vi "SBA-5_command case_v2.vi"(6 "Valve control":bool=TRUE, 7 "Case":T1(ring), 8 "error in (no error)":errorcluster, 9 "Val 2":dbl, 10 "Val 1":i32, 11 "VISA resource name":refnum<visa-resource-name>) -> (0 "error out":errorcluster, 1 "bytes out":u32, 2 "StringFromSBA-5":string, 3 "dup VISA resource name":refnum<visa-resource-name>)   [LabVIEW 2016]
uses:
  <vilib>/Instr/_visa.llb/VISA Flush IO Buffer Mask.ctl
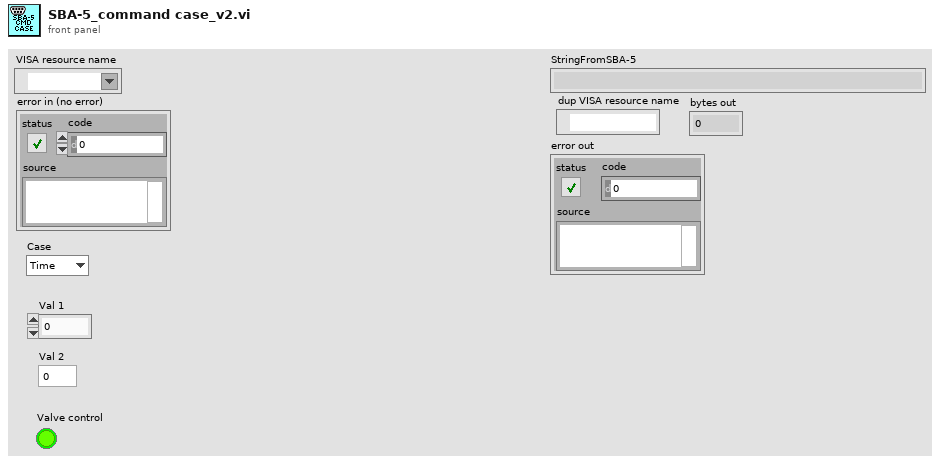
[diagram p1: front panel]
types:
  T1 = enum16{"Time", "Zero", "Poll", "Read Buffer", "Set Stream", "Set Poll", "Pump On", "Pump Off", "Set Zero Timing", "Set CO2 Avg.", "Set Measument Format", "Startup Zero Off", "Statup Zero On", "Short Zero Duration", "Set Scaling Factor", "Set Dec Points", "Set Low CO2 Alarm", "Set Analog Output Type", "Set Analog Output Scaling", "Set Data Valid Pin I/O", "Save Current Settings", "Restore Default Settings", "Display Current Settings", "Medium Zero Duration", "Long Zero Duration"}
  T2 = typedef "VISA Flush IO Buffer Mask.ctl" = u16
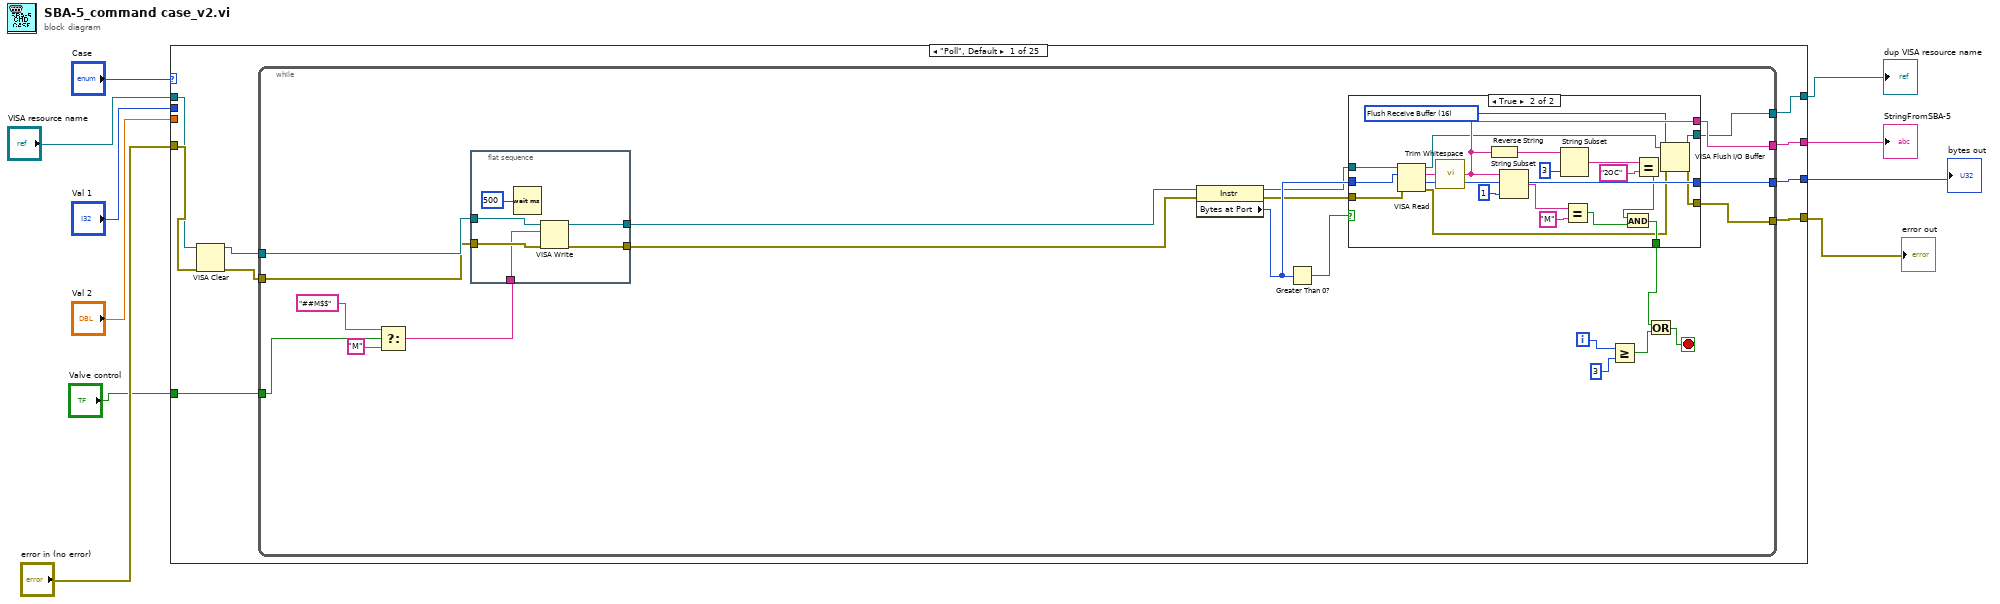
[diagram p0: block diagram]
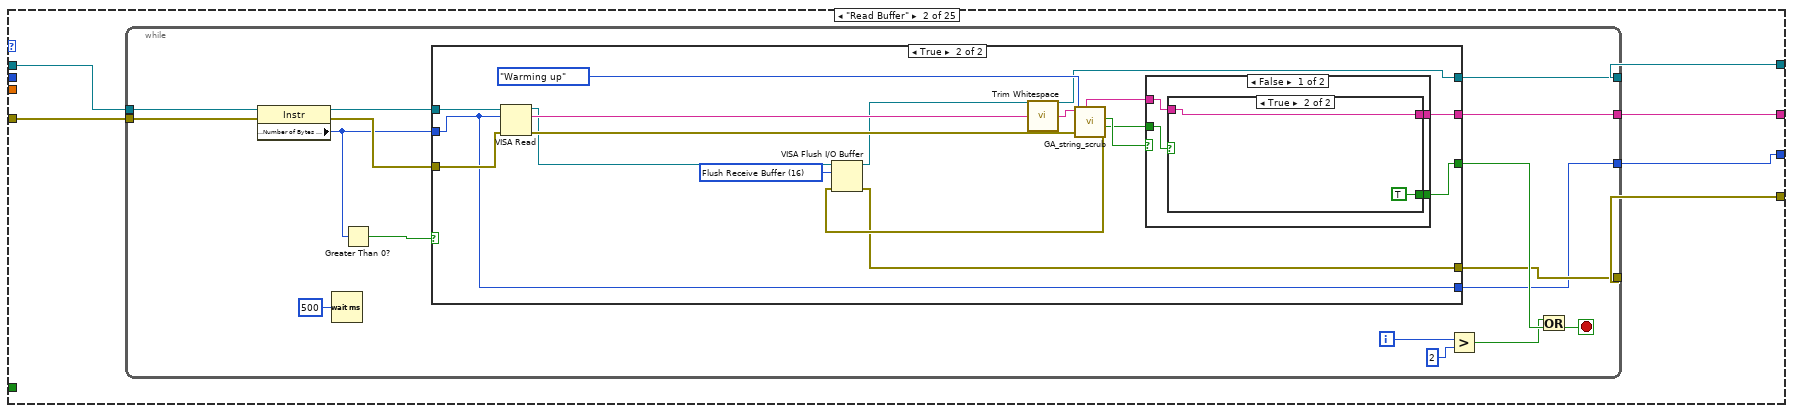
[diagram p3: hidden frame]
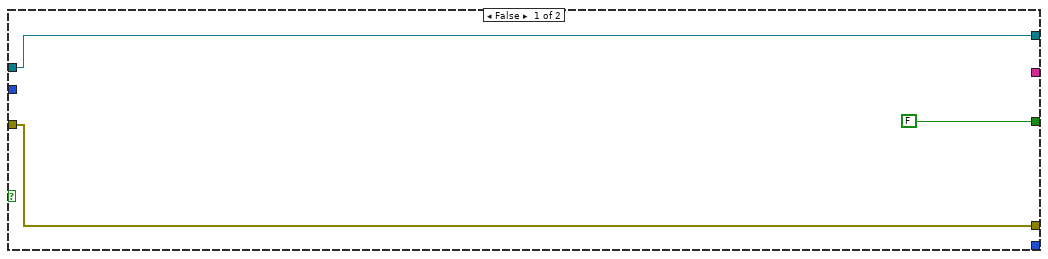
[diagram p4: hidden frame]
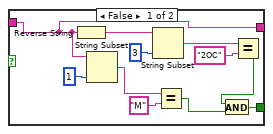
[diagram p5: hidden frame]
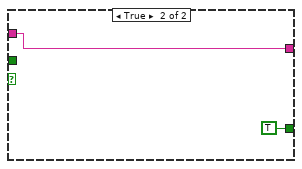
[diagram p6: hidden frame]
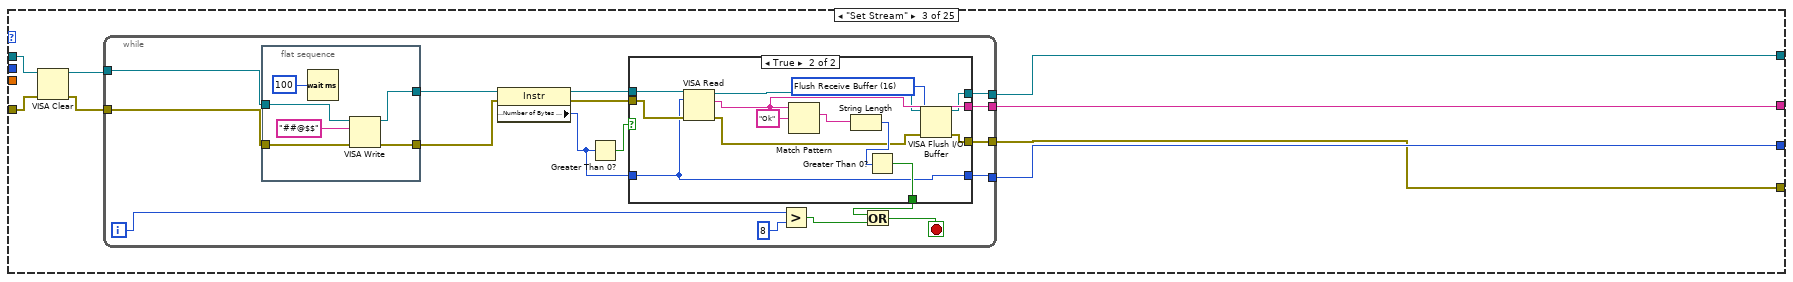
[diagram p7: hidden frame]
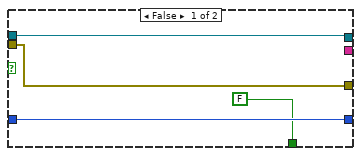
[diagram p8: hidden frame]
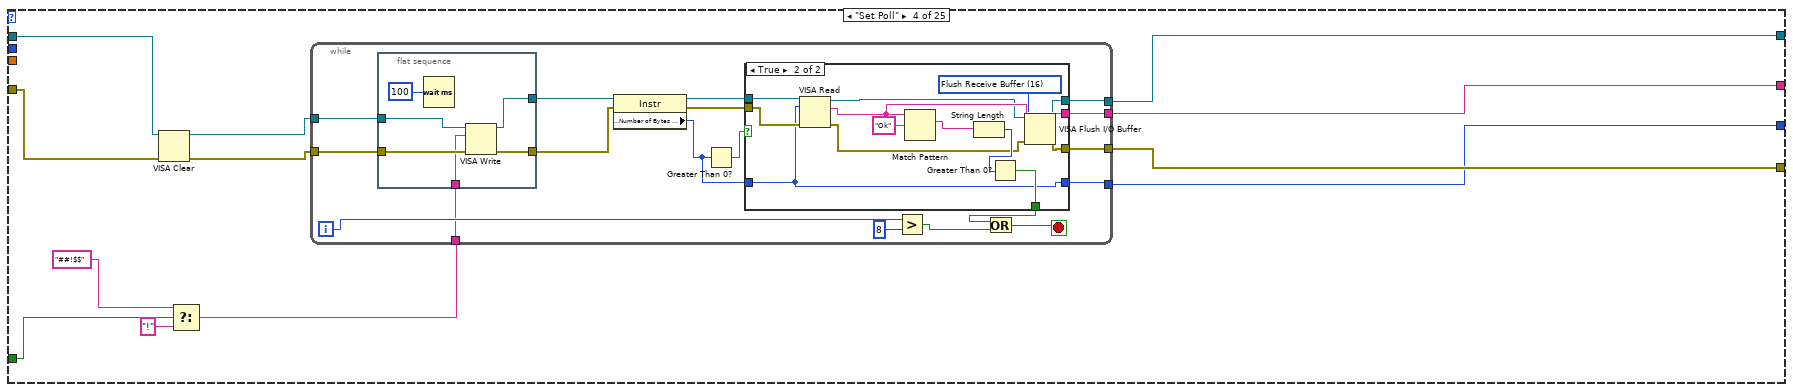
[diagram p9: hidden frame]
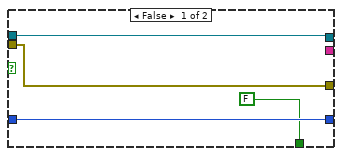
[diagram p10: hidden frame]
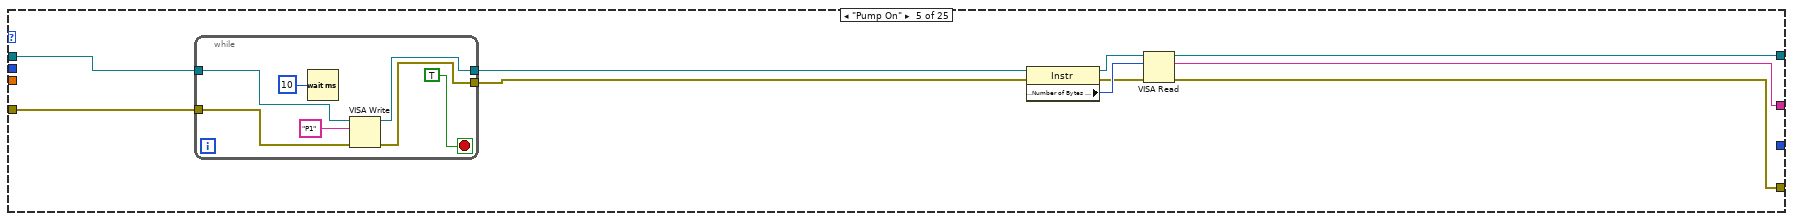
[diagram p11: hidden frame]
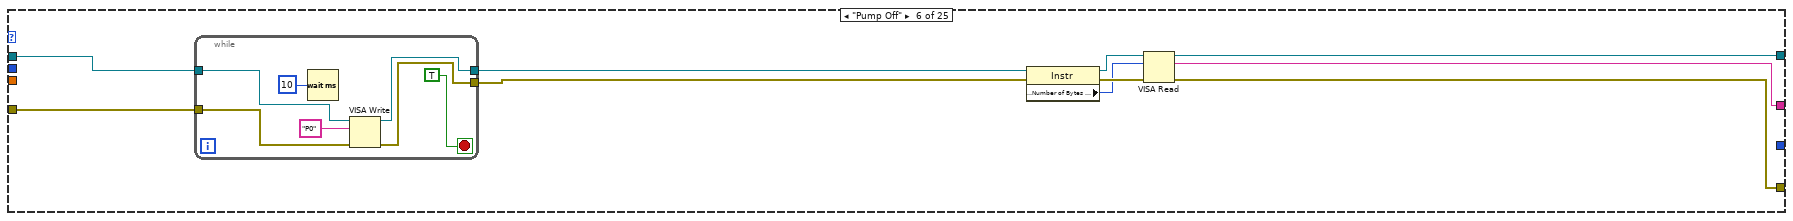
[diagram p12: hidden frame]
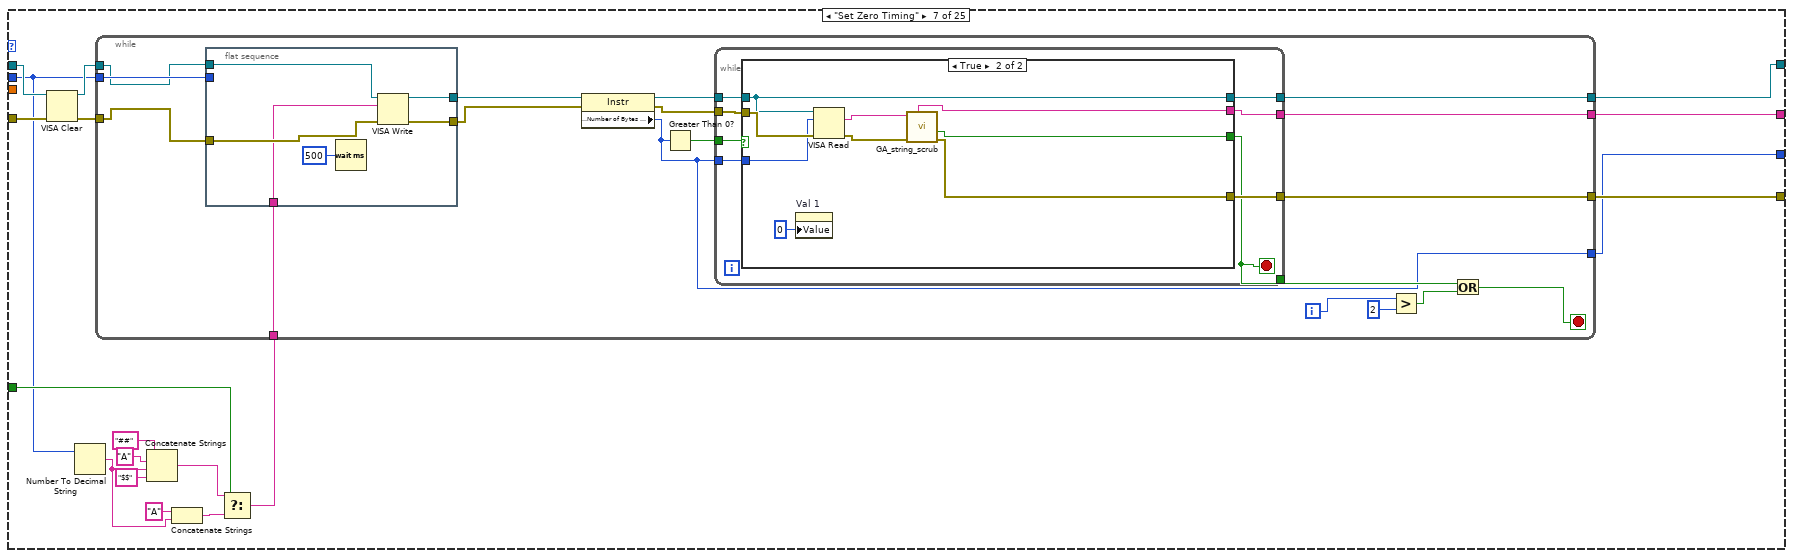
[diagram p13: hidden frame]
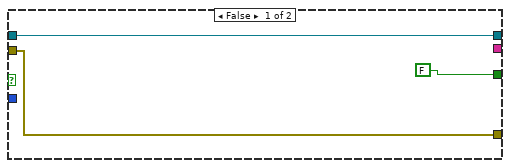
[diagram p14: hidden frame]
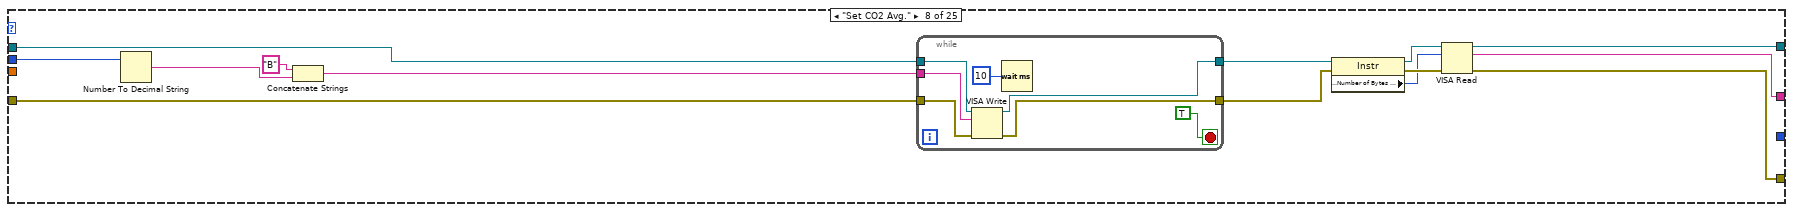
[diagram p15: hidden frame]
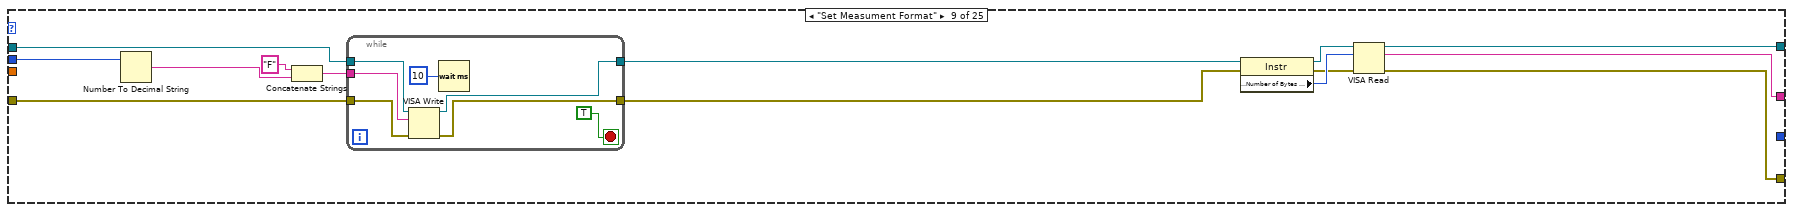
[diagram p16: hidden frame]
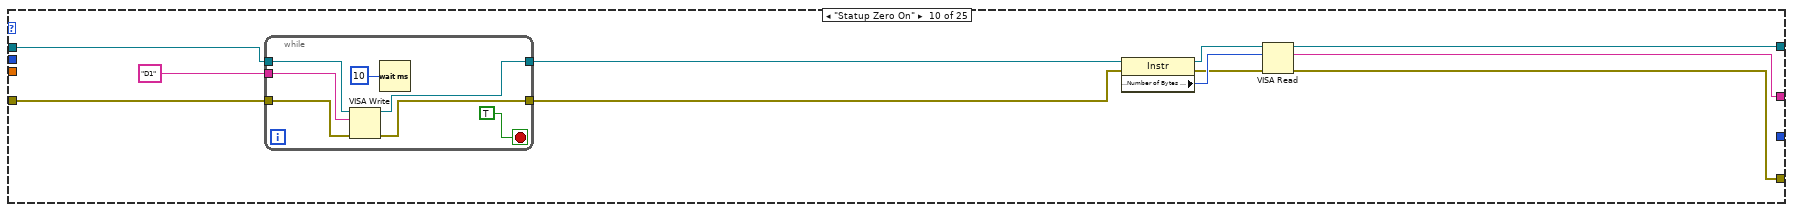
[diagram p17: hidden frame]
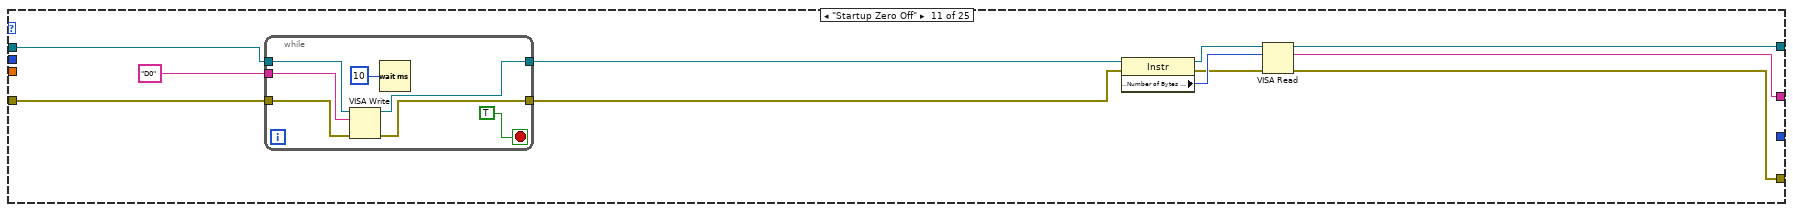
[diagram p18: hidden frame]
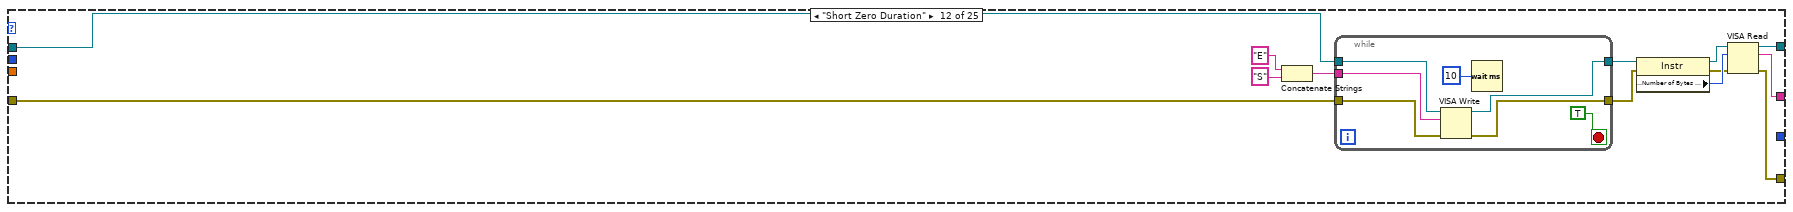
[diagram p19: hidden frame]
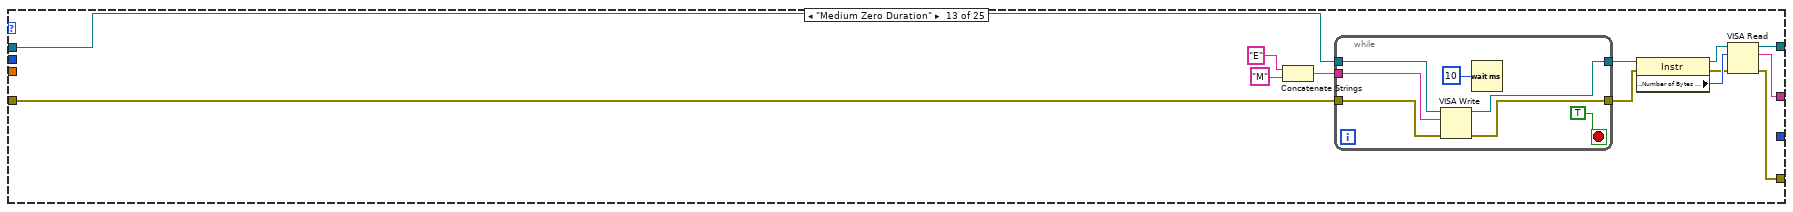
[diagram p20: hidden frame]
diagram:
  n1 = case shown="\"Poll\", Default" "Case" {
    tunnel: "VISA resource name" -> [w13 w76 w133 w185 w237 w254 w278 w333 w354 w376 w393 w412 w432 w452 w472 w493 w513 w535 w562 w580 w602 w619 w637 w652 w675]
    tunnel: "error in (no error)" -> [w15 w75 w135 w184 w236 w253 w284 w332 w353 w375 w392 w411 w431 w451 w471 w492 w512 w534 w561 w579 w601 w618 w636 w651 w674]
    tunnel: [w19 w74 w139 w191 w235 w252 w283 w331 w352 w374 w391 w410 w430 w450 w470 w491 w511 w533 w560 w578 w600 w617 w635 w653 w673] -> w4
    tunnel: [w17 w73 w137 w189 w234 w251 w282 w329 w351 w373 w390 w408 w428 w448 w469 w490 w510 w532 w559 w577 w598 w616 w634 w654 w671] -> w3
    tunnel: [w18 w72 w136 w190 w233 w250 w280 w330 w350 w372 w389 w409 w429 w449 w468 w489 w509 w531 w558 w576 w599 w615 w633 w655 w670] -> w5
    tunnel: "Val 2" -> [_ _ _ _ _ _ _ _ _ _ _ _ _ _ w467 _ _ _ w563 _ _ _ _ _ _]
    tunnel: "Val 1" -> [_ _ _ _ _ _ w271 w334 w355 _ _ _ _ _ _ w488 w514 w530 w556 w581 _ _ _ _ _]
    tunnel: [w16 w71 w138 w188 _ _ w281 _ _ _ _ _ _ _ _ _ _ _ _ _ _ _ _ _ w672] -> w2
    tunnel: "Valve control" -> [w11 _ _ w183 _ _ w276 _ _ _ _ _ _ _ _ _ _ _ _ _ _ _ _ _ _]
    frame "Poll", Default {
      n2 = VISA Clear(VISA resource name=w13, error in (no error)=w15) -> (VISA resource name out=w12:refnum<visa-resource-name>, error out=w14:errorcluster)
      n3 = while {
        tunnel: [w31] -> w19
        tunnel: [w30] -> w17
        tunnel: w12 -> [w40]
        tunnel: w14 -> [w39]
        tunnel: [w32] -> w18
        tunnel: [w29] -> w16
        tunnel: w11 -> [w23]
        i -> [w28]
        stop <- w24 stop-if-true
        n4 = Select(t="##M$$" ("write buffer"), s=w23, f="M") -> (s? t:f=w21:string)
        n5 = flat-sequence {
          tunnel: w40 -> [w70]
          tunnel: w39 -> [w69]
          tunnel: [w68] -> w38
          tunnel: [w67] -> w37
          tunnel: w21 -> [w65]
          frame #0 {
            n6 = Wait (ms)(milliseconds to wait=u32 500) -> ()  [unwired: 1 out]
            n7 = VISA Write(VISA resource name=w70, write buffer=w65, error in (no error)=w69) -> (VISA resource name out=w68:refnum<visa-resource-name>, error out=w67:errorcluster)  [unwired: 1 out]
          }
        }
        n8 = property class="Instr"(reference=w38, error in=w37) -> (reference out=w34:refnum<visa-resource-name>, error out=w33:errorcluster, "Bytes at Port"=w35:u32)
        n9 = Greater Than 0?(x=w35) -> (x > 0?=w36:bool)
        n10 = case shown="True" w36 {
          tunnel: [_ w52] -> w32
          tunnel: [w41 w64] -> w29
          tunnel: [w43 w45] -> w31
          tunnel: [w42 w44] -> w30
          tunnel: w33 -> [w42 w63]
          tunnel: w35 -> [w41 w62]
          tunnel: w34 -> [w43 w61]
          tunnel: [_ w49] -> w26
          frame False {
          }
          frame True {
            w46 = T2 16 items=["Flush Receive Buffer"=16, "Write Transmit Buffer to Device"=32, "Flush Receive Buffer (No I/O)"=64, "Flush Transmit Buffer"=128] ("Mask")
            n11 = VISA Read(VISA resource name=w61, byte count=w62, error in (no error)=w63) -> (VISA resource name out=w48:refnum<visa-resource-name>, read buffer=w57:string, return count=w64:u32, error out=w47:errorcluster)
            n12 = call <vilib>:"Trim Whitespace.vi"("string"=w57) -> ("trimmed string"=w52:string)  [unwired: 1 in]
            n13 = Reverse String(1:w52) -> (0:w56:string)
            n14 = String Subset(string=w52, length (rest)=1 ("length (rest)")) -> (substring=w59:string)  [unwired: 1 in]
            n15 = String Subset(string=w56, length (rest)=3 ("length (rest)")) -> (substring=w54:string)  [unwired: 1 in]
            n16 = Equal?(x=w59, y="M") -> (x = y?=w51:bool)
            n17 = Equal?(x=w54, y="2OC") -> (x = y?=w50:bool)
            n18 = And(x=w50, y=w51) -> (x .and. y?=w49:bool)
            n19 = VISA Flush I/O Buffer(VISA resource name=w48, mask (16)=w46, error in (no error)=w47) -> (VISA resource name out=w45:refnum<visa-resource-name>, error out=w44:errorcluster)
          }
        }
        n20 = Greater Or Equal?(x=w28, y=3) -> (x >= y?=w25:bool)
        n21 = Or(x=w26, y=w25) -> (x .or. y?=w24:bool)
      }
    }
    frame "Read Buffer" {
      n22 = while {
        tunnel: w76 -> [w92]
        tunnel: w75 -> [w91]
        tunnel: [w85] -> w74
        tunnel: [w84] -> w73
        tunnel: [w78] -> w72
        tunnel: [w77] -> w71
        i -> [w81]
        stop <- w83 stop-if-true
        n23 = property class="Instr"(reference=w92, error in=w91) -> (reference out=w90:refnum<visa-resource-name>, error out=w89:errorcluster, "Serial Settings:Number of Bytes at Serial Port"=w88:u32)
        n24 = Wait (ms)(milliseconds to wait=u32 500) -> ()  [unwired: 1 out]
        n25 = Greater Than 0?(x=w88) -> (x > 0?=w87:bool)
        n26 = case shown="True" w87 {
          tunnel: w90 -> [w95 w112]
          tunnel: w89 -> [w94 w111]
          tunnel: w88 -> [_ w101]
          tunnel: [w95 w97] -> w85
          tunnel: [w94 w98] -> w84
          tunnel: [FALSE w103] -> w86
          tunnel: [_ w102] -> w78
          tunnel: [_ w101] -> w77
          frame False {
          }
          frame True {
            w96 = T2 16 items=["Flush Receive Buffer"=16, "Write Transmit Buffer to Device"=32, "Flush Receive Buffer (No I/O)"=64, "Flush Transmit Buffer"=128] ("Mask")
            n27 = VISA Read(VISA resource name=w112, byte count=w101, error in (no error)=w111) -> (VISA resource name out=w100:refnum<visa-resource-name>, read buffer=w110:string, error out=w107:errorcluster)  [unwired: 1 out]
            n28 = call <vilib>:"Trim Whitespace.vi"("string"=w110) -> ("trimmed string"=w109:string)  [unwired: 1 in]
            n29 = call "GA_string_scrub.vi"("error in (no error)"=w107, "opMode"=enum16{"Warming up", "Runtime"}."Warming up", "input"=w109) -> ("error out"=w99:errorcluster, "Zeroing"=w105:bool, "Warming up"=w106:bool, "output string"=w104:string)  [unwired: 1 in, 4 out]
            n30 = VISA Flush I/O Buffer(VISA resource name=w100, mask (16)=w96, error in (no error)=w99) -> (VISA resource name out=w97:refnum<visa-resource-name>, error out=w98:errorcluster)
            n31 = case shown="False" w106 {
              tunnel: w105 -> [w116 _]
              tunnel: w104 -> [w115 w131]
              tunnel: [w114 TRUE] -> w103
              tunnel: [w113 w131] -> w102
              frame False {
                n32 = case shown="True" w116 {
                  tunnel: w115 -> [w117 w129]
                  tunnel: [w118 TRUE] -> w114
                  tunnel: [w117 w129] -> w113
                  frame False {
                    n33 = Reverse String(1:w117) -> (0:w123:string)
                    n34 = String Subset(string=w117, length (rest)=1 ("length (rest)")) -> (substring=w121:string)  [unwired: 1 in]
                    n35 = String Subset(string=w123, length (rest)=3 ("length (rest)")) -> (substring=w125:string)  [unwired: 1 in]
                    n36 = Equal?(x=w121, y="M") -> (x = y?=w119:bool)
                    n37 = Equal?(x=w125, y="2OC") -> (x = y?=w127:bool)
                    n38 = And(x=w127, y=w119) -> (x .and. y?=w118:bool)
                  }
                  frame True {
                  }
                }
              }
              frame True {
              }
            }
          }
        }
        n39 = Greater?(x=w81, y=2) -> (0:w79:bool)
        n40 = Or(x=w79, y=w86) -> (x .or. y?=w83:bool)
      }
    }
    frame "Set Stream" {
      n41 = VISA Clear(VISA resource name=w133, error in (no error)=w135) -> (VISA resource name out=w132:refnum<visa-resource-name>, error out=w134:errorcluster)
      n42 = while {
        tunnel: w132 -> [w156]
        tunnel: w134 -> [w155]
        tunnel: [w148] -> w139
        tunnel: [w147] -> w137
        tunnel: [w146] -> w138
        tunnel: [w145] -> w136
        i -> [w142]
        stop <- w144 stop-if-true
        n43 = flat-sequence {
          tunnel: w156 -> [w178]
          tunnel: w155 -> [w177]
          tunnel: [w175] -> w154
          tunnel: [w174] -> w153
          frame #0 {
            n44 = Wait (ms)(milliseconds to wait=u32 100) -> ()  [unwired: 1 out]
            n45 = VISA Write(VISA resource name=w178, write buffer="##@$$", error in (no error)=w177) -> (VISA resource name out=w175:refnum<visa-resource-name>, error out=w174:errorcluster)  [unwired: 1 out]
          }
        }
        n46 = property class="Instr"(reference=w154, error in=w153) -> (reference out=w151:refnum<visa-resource-name>, error out=w150:errorcluster, "Serial Settings:Number of Bytes at Serial Port"=w149:u32)
        n47 = Greater Than 0?(x=w149) -> (x > 0?=w152:bool)
        n48 = case shown="True" w152 {
          tunnel: w151 -> [w160 w173]
          tunnel: w150 -> [w159 w172]
          tunnel: w149 -> [w158 w167]
          tunnel: [FALSE w168] -> w143
          tunnel: [w160 w164] -> w148
          tunnel: [w159 w162] -> w147
          tunnel: [w158 w167] -> w146
          tunnel: [_ w166] -> w145
          frame False {
          }
          frame True {
            w161 = T2 16 items=["Flush Receive Buffer"=16, "Write Transmit Buffer to Device"=32, "Flush Receive Buffer (No I/O)"=64, "Flush Transmit Buffer"=128] ("Mask")
            n49 = VISA Read(VISA resource name=w173, byte count=w167, error in (no error)=w172) -> (VISA resource name out=w165:refnum<visa-resource-name>, read buffer=w166:string, error out=w163:errorcluster)  [unwired: 1 out]
            n50 = Match Pattern(string=w166, regular expression="Ok") -> (match substring=w170:string)  [unwired: 1 in, 3 out]
            n51 = String Length(string=w170) -> (length=w169:i32)
            n52 = Greater Than 0?(x=w169) -> (x > 0?=w168:bool)
            n53 = VISA Flush I/O Buffer(VISA resource name=w165, mask (16)=w161, error in (no error)=w163) -> (VISA resource name out=w164:refnum<visa-resource-name>, error out=w162:errorcluster)
          }
        }
        n54 = Greater?(x=w142, y=8) -> (0:w140:bool)
        n55 = Or(x=w143, y=w140) -> (x .or. y?=w144:bool)
      }
    }
    frame "Set Poll" {
      n56 = VISA Clear(VISA resource name=w185, error in (no error)=w184) -> (VISA resource name out=w187:refnum<visa-resource-name>, error out=w186:errorcluster)
      n57 = Select(t="##!$$" ("write buffer"), s=w183, f="!") -> (s? t:f=w180:string)
      n58 = while {
        tunnel: [w203] -> w191
        tunnel: [w202] -> w189
        tunnel: [w201] -> w188
        tunnel: [w200] -> w190
        tunnel: w187 -> [w194]
        tunnel: w186 -> [w193]
        tunnel: w180 -> [w192]
        i -> [w197]
        stop <- w199 stop-if-true
        n59 = flat-sequence {
          tunnel: [w231] -> w209
          tunnel: [w230] -> w208
          tunnel: w194 -> [w229]
          tunnel: w193 -> [w228]
          tunnel: w192 -> [w227]
          frame #0 {
            n60 = Wait (ms)(milliseconds to wait=u32 100) -> ()  [unwired: 1 out]
            n61 = VISA Write(VISA resource name=w229, write buffer=w227, error in (no error)=w228) -> (VISA resource name out=w231:refnum<visa-resource-name>, error out=w230:errorcluster)  [unwired: 1 out]
          }
        }
        n62 = property class="Instr"(reference=w209, error in=w208) -> (reference out=w206:refnum<visa-resource-name>, error out=w205:errorcluster, "Serial Settings:Number of Bytes at Serial Port"=w204:u32)
        n63 = Greater Than 0?(x=w204) -> (x > 0?=w207:bool)
        n64 = case shown="True" w207 {
          tunnel: w206 -> [w213 w226]
          tunnel: w205 -> [w212 w225]
          tunnel: w204 -> [w211 w220]
          tunnel: [FALSE w221] -> w198
          tunnel: [w213 w217] -> w203
          tunnel: [w212 w215] -> w202
          tunnel: [w211 w220] -> w201
          tunnel: [_ w219] -> w200
          frame False {
          }
          frame True {
            w214 = T2 16 items=["Flush Receive Buffer"=16, "Write Transmit Buffer to Device"=32, "Flush Receive Buffer (No I/O)"=64, "Flush Transmit Buffer"=128] ("Mask")
            n65 = VISA Read(VISA resource name=w226, byte count=w220, error in (no error)=w225) -> (VISA resource name out=w218:refnum<visa-resource-name>, read buffer=w219:string, error out=w216:errorcluster)  [unwired: 1 out]
            n66 = Match Pattern(string=w219, regular expression="Ok") -> (match substring=w223:string)  [unwired: 1 in, 3 out]
            n67 = String Length(string=w223) -> (length=w222:i32)
            n68 = Greater Than 0?(x=w222) -> (x > 0?=w221:bool)
            n69 = VISA Flush I/O Buffer(VISA resource name=w218, mask (16)=w214, error in (no error)=w216) -> (VISA resource name out=w217:refnum<visa-resource-name>, error out=w215:errorcluster)
          }
        }
        n70 = Greater?(x=w197, y=8) -> (0:w195:bool)
        n71 = Or(x=w198, y=w195) -> (x .or. y?=w199:bool)
      }
    }
    frame "Pump On" {
      n72 = while {
        tunnel: [w248] -> w242
        tunnel: [w247] -> w241
        tunnel: w237 -> [w246]
        tunnel: w236 -> [w245]
        stop <- TRUE stop-if-true
        n73 = Wait (ms)(milliseconds to wait=u32 10) -> ()  [unwired: 1 out]
        n74 = VISA Write(VISA resource name=w246, write buffer="P1" ("string"), error in (no error)=w245) -> (VISA resource name out=w248:refnum<visa-resource-name>, error out=w247:errorcluster)  [unwired: 1 out]
      }
      n75 = property class="Instr"(reference=w242, error in=w241) -> (reference out=w239:refnum<visa-resource-name>, error out=w238:errorcluster, "Serial Settings:Number of Bytes at Serial Port"=w240:u32)
      n76 = VISA Read(VISA resource name=w239, byte count=w240, error in (no error)=w238) -> (VISA resource name out=w235:refnum<visa-resource-name>, read buffer=w233:string, error out=w234:errorcluster)  [unwired: 1 out]
    }
    frame "Pump Off" {
      n77 = while {
        tunnel: [w265] -> w256
        tunnel: [w264] -> w255
        tunnel: w254 -> [w262]
        tunnel: w253 -> [w261]
        stop <- TRUE stop-if-true
        n78 = Wait (ms)(milliseconds to wait=u32 10) -> ()  [unwired: 1 out]
        n79 = VISA Write(VISA resource name=w262, write buffer="P0" ("string"), error in (no error)=w261) -> (VISA resource name out=w264:refnum<visa-resource-name>, error out=w265:errorcluster)  [unwired: 1 out]
      }
      n80 = property class="Instr"(reference=w255, error in=w256) -> (reference out=w258:refnum<visa-resource-name>, error out=w259:errorcluster, "Serial Settings:Number of Bytes at Serial Port"=w257:u32)
      n81 = VISA Read(VISA resource name=w258, byte count=w257, error in (no error)=w259) -> (VISA resource name out=w252:refnum<visa-resource-name>, read buffer=w250:string, error out=w251:errorcluster)  [unwired: 1 out]
    }
    frame "Set Zero Timing" {
      n82 = VISA Clear(VISA resource name=w278, error in (no error)=w284) -> (VISA resource name out=w277:refnum<visa-resource-name>, error out=w279:errorcluster)
      n83 = Number To Decimal String(number=w271) -> (decimal integer string=w267:string)  [unwired: 1 in]
      n84 = Concatenate Strings("##" ("string"), "A", w267, "$$" ("string")) -> (w272:string)
      n85 = Concatenate Strings("A" ("string"), w267) -> (w269:string)
      n86 = Select(t=w272, s=w276, f=w269) -> (s? t:f=w270:string)
      n87 = while {
        tunnel: w271 -> [w302]
        tunnel: w277 -> [w287]
        tunnel: w279 -> [w286]
        tunnel: [w291] -> w283
        tunnel: [w290] -> w282
        tunnel: [w289] -> w281
        tunnel: [w288] -> w280
        tunnel: w270 -> [w285]
        i -> [w295]
        stop <- w292 stop-if-true
        n88 = flat-sequence {
          tunnel: w302 -> [_]
          tunnel: [w327] -> w301
          tunnel: [w326] -> w300
          tunnel: w287 -> [w325]
          tunnel: w286 -> [w324]
          tunnel: w285 -> [w323]
          frame #0 {
            n89 = Wait (ms)(milliseconds to wait=u32 500) -> ()  [unwired: 1 out]
            n90 = VISA Write(VISA resource name=w325, write buffer=w323, error in (no error)=w324) -> (VISA resource name out=w327:refnum<visa-resource-name>, error out=w326:errorcluster)  [unwired: 1 out]
          }
        }
        n91 = property class="Instr"(reference=w301, error in=w300) -> (reference out=w298:refnum<visa-resource-name>, error out=w297:errorcluster, "Serial Settings:Number of Bytes at Serial Port"=w289:u32)
        n92 = Greater Than 0?(x=w289) -> (x > 0?=w299:bool)
        n93 = while {
          tunnel: w299 -> [w310]
          tunnel: w298 -> [w309]
          tunnel: w297 -> [w308]
          tunnel: [w303] -> w296
          tunnel: [w307] -> w291
          tunnel: [w306] -> w290
          tunnel: w289 -> [w305]
          tunnel: [w304] -> w288
          stop <- w303 stop-if-true
          n94 = case shown="True" w310 {
            tunnel: w309 -> [w312 w320]
            tunnel: w308 -> [w311 w322]
            tunnel: w305 -> [_ w321]
            tunnel: [FALSE w316] -> w303
            tunnel: [w312 w320] -> w307
            tunnel: [w311 w314] -> w306
            tunnel: [_ w317] -> w304
            frame False {
            }
            frame True {
              n95 = property on="Val 1" class="DigNum (strict)"("Value"=0 ("Val 1")) -> ()  [unwired: 2 in, 2 out]
              n96 = VISA Read(VISA resource name=w320, byte count=w321, error in (no error)=w322) -> (read buffer=w318:string, error out=w315:errorcluster)  [unwired: 2 out]
              n97 = call "GA_string_scrub.vi"("error in (no error)"=w315, "input"=w318) -> ("error out"=w314:errorcluster, "Zeroing"=w316:bool, "output string"=w317:string)  [unwired: 2 in, 5 out]
            }
          }
        }
        n98 = Greater?(x=w295, y=2) -> (0:w293:bool)
        n99 = Or(x=w296, y=w293) -> (x .or. y?=w292:bool)
      }
    }
    frame "Set CO2 Avg." {
      n100 = Number To Decimal String(number=w334) -> (decimal integer string=w341:string)  [unwired: 1 in]
      n101 = Concatenate Strings("B", w341) -> (w342:string)
      n102 = while {
        tunnel: w342 -> [w349]
        tunnel: [w348] -> w336
        tunnel: [w347] -> w335
        tunnel: w333 -> [w345]
        tunnel: w332 -> [w344]
        stop <- TRUE stop-if-true
        n103 = VISA Write(VISA resource name=w345, write buffer=w349, error in (no error)=w344) -> (VISA resource name out=w347:refnum<visa-resource-name>, error out=w348:errorcluster)  [unwired: 1 out]
        n104 = Wait (ms)(milliseconds to wait=u32 10) -> ()  [unwired: 1 out]
      }
      n105 = property class="Instr"(reference=w335, error in=w336) -> (reference out=w338:refnum<visa-resource-name>, error out=w339:errorcluster, "Serial Settings:Number of Bytes at Serial Port"=w337:u32)
      n106 = VISA Read(VISA resource name=w338, byte count=w337, error in (no error)=w339) -> (VISA resource name out=w331:refnum<visa-resource-name>, read buffer=w330:string, error out=w329:errorcluster)  [unwired: 1 out]
    }
    frame "Set Measument Format" {
      n107 = Number To Decimal String(number=w355) -> (decimal integer string=w357:string)  [unwired: 1 in]
      n108 = Concatenate Strings("F", w357) -> (w356:string)
      n109 = while {
        tunnel: [w369] -> w363
        tunnel: [w368] -> w362
        tunnel: w356 -> [w367]
        tunnel: w354 -> [w366]
        tunnel: w353 -> [w365]
        stop <- TRUE stop-if-true
        n110 = VISA Write(VISA resource name=w366, write buffer=w367, error in (no error)=w365) -> (VISA resource name out=w369:refnum<visa-resource-name>, error out=w368:errorcluster)  [unwired: 1 out]
        n111 = Wait (ms)(milliseconds to wait=u32 10) -> ()  [unwired: 1 out]
      }
      n112 = property class="Instr"(reference=w363, error in=w362) -> (reference out=w360:refnum<visa-resource-name>, error out=w359:errorcluster, "Serial Settings:Number of Bytes at Serial Port"=w361:u32)
      n113 = VISA Read(VISA resource name=w360, byte count=w361, error in (no error)=w359) -> (VISA resource name out=w352:refnum<visa-resource-name>, read buffer=w350:string, error out=w351:errorcluster)  [unwired: 1 out]
    }
    frame "Statup Zero On" {
      n114 = while {
        tunnel: [w387] -> w381
        tunnel: [w386] -> w380
        tunnel: w376 -> [w385]
        tunnel: w375 -> [w384]
        tunnel: "D1" -> [w383]
        stop <- TRUE stop-if-true
        n115 = VISA Write(VISA resource name=w385, write buffer=w383, error in (no error)=w384) -> (VISA resource name out=w387:refnum<visa-resource-name>, error out=w386:errorcluster)  [unwired: 1 out]
        n116 = Wait (ms)(milliseconds to wait=u32 10) -> ()  [unwired: 1 out]
      }
      n117 = property class="Instr"(reference=w381, error in=w380) -> (reference out=w378:refnum<visa-resource-name>, error out=w377:errorcluster, "Serial Settings:Number of Bytes at Serial Port"=w379:u32)
      n118 = VISA Read(VISA resource name=w378, byte count=w379, error in (no error)=w377) -> (VISA resource name out=w374:refnum<visa-resource-name>, read buffer=w372:string, error out=w373:errorcluster)  [unwired: 1 out]
    }
    frame "Startup Zero Off" {
      n119 = while {
        tunnel: [w405] -> w399
        tunnel: [w404] -> w398
        tunnel: "D0" -> [w403]
        tunnel: w393 -> [w402]
        tunnel: w392 -> [w401]
        stop <- TRUE stop-if-true
        n120 = VISA Write(VISA resource name=w402, write buffer=w403, error in (no error)=w401) -> (VISA resource name out=w405:refnum<visa-resource-name>, error out=w404:errorcluster)  [unwired: 1 out]
        n121 = Wait (ms)(milliseconds to wait=u32 10) -> ()  [unwired: 1 out]
      }
      n122 = property class="Instr"(reference=w399, error in=w398) -> (reference out=w396:refnum<visa-resource-name>, error out=w395:errorcluster, "Serial Settings:Number of Bytes at Serial Port"=w397:u32)
      n123 = VISA Read(VISA resource name=w396, byte count=w397, error in (no error)=w395) -> (VISA resource name out=w391:refnum<visa-resource-name>, read buffer=w389:string, error out=w390:errorcluster)  [unwired: 1 out]
    }
    frame "Short Zero Duration" {
      n124 = Concatenate Strings("E", "S" ("string")) -> (w413:string)
      n125 = while {
        tunnel: [w425] -> w419
        tunnel: [w424] -> w418
        tunnel: w413 -> [w423]
        tunnel: w412 -> [w422]
        tunnel: w411 -> [w421]
        stop <- TRUE stop-if-true
        n126 = VISA Write(VISA resource name=w422, write buffer=w423, error in (no error)=w421) -> (VISA resource name out=w425:refnum<visa-resource-name>, error out=w424:errorcluster)  [unwired: 1 out]
        n127 = Wait (ms)(milliseconds to wait=u32 10) -> ()  [unwired: 1 out]
      }
      n128 = property class="Instr"(reference=w419, error in=w418) -> (reference out=w416:refnum<visa-resource-name>, error out=w415:errorcluster, "Serial Settings:Number of Bytes at Serial Port"=w417:u32)
      n129 = VISA Read(VISA resource name=w416, byte count=w417, error in (no error)=w415) -> (VISA resource name out=w410:refnum<visa-resource-name>, read buffer=w409:string, error out=w408:errorcluster)  [unwired: 1 out]
    }
    frame "Medium Zero Duration" {
      n130 = Concatenate Strings("E", "M" ("string")) -> (w433:string)
      n131 = while {
        tunnel: [w445] -> w439
        tunnel: [w444] -> w438
        tunnel: w433 -> [w443]
        tunnel: w432 -> [w442]
        tunnel: w431 -> [w441]
        stop <- TRUE stop-if-true
        n132 = VISA Write(VISA resource name=w442, write buffer=w443, error in (no error)=w441) -> (VISA resource name out=w445:refnum<visa-resource-name>, error out=w444:errorcluster)  [unwired: 1 out]
        n133 = Wait (ms)(milliseconds to wait=u32 10) -> ()  [unwired: 1 out]
      }
      n134 = property class="Instr"(reference=w439, error in=w438) -> (reference out=w436:refnum<visa-resource-name>, error out=w435:errorcluster, "Serial Settings:Number of Bytes at Serial Port"=w437:u32)
      n135 = VISA Read(VISA resource name=w436, byte count=w437, error in (no error)=w435) -> (VISA resource name out=w430:refnum<visa-resource-name>, read buffer=w429:string, error out=w428:errorcluster)  [unwired: 1 out]
    }
    frame "Long Zero Duration" {
      n136 = Concatenate Strings("E", "L" ("string")) -> (w453:string)
      n137 = while {
        tunnel: [w465] -> w459
        tunnel: [w464] -> w458
        tunnel: w453 -> [w463]
        tunnel: w452 -> [w462]
        tunnel: w451 -> [w461]
        stop <- TRUE stop-if-true
        n138 = VISA Write(VISA resource name=w462, write buffer=w463, error in (no error)=w461) -> (VISA resource name out=w465:refnum<visa-resource-name>, error out=w464:errorcluster)  [unwired: 1 out]
        n139 = Wait (ms)(milliseconds to wait=u32 10) -> ()  [unwired: 1 out]
      }
      n140 = property class="Instr"(reference=w459, error in=w458) -> (reference out=w456:refnum<visa-resource-name>, error out=w455:errorcluster, "Serial Settings:Number of Bytes at Serial Port"=w457:u32)
      n141 = VISA Read(VISA resource name=w456, byte count=w457, error in (no error)=w455) -> (VISA resource name out=w450:refnum<visa-resource-name>, read buffer=w449:string, error out=w448:errorcluster)  [unwired: 1 out]
    }
    frame "Set Scaling Factor" {
      n142 = Number To Decimal String(number=w467) -> (decimal integer string=w474:string)  [unwired: 1 in]
      n143 = Concatenate Strings("U", w474) -> (w473:string)
      n144 = while {
        tunnel: [w486] -> w480
        tunnel: [w485] -> w479
        tunnel: w473 -> [w484]
        tunnel: w472 -> [w483]
        tunnel: w471 -> [w482]
        stop <- TRUE stop-if-true
        n145 = VISA Write(VISA resource name=w483, write buffer=w484, error in (no error)=w482) -> (VISA resource name out=w486:refnum<visa-resource-name>, error out=w485:errorcluster)  [unwired: 1 out]
        n146 = Wait (ms)(milliseconds to wait=u32 10) -> ()  [unwired: 1 out]
      }
      n147 = property class="Instr"(reference=w480, error in=w479) -> (reference out=w477:refnum<visa-resource-name>, error out=w476:errorcluster, "Serial Settings:Number of Bytes at Serial Port"=w478:u32)
      n148 = VISA Read(VISA resource name=w477, byte count=w478, error in (no error)=w476) -> (VISA resource name out=w470:refnum<visa-resource-name>, read buffer=w468:string, error out=w469:errorcluster)  [unwired: 1 out]
    }
    frame "Set Dec Points" {
      n149 = Number To Decimal String(number=w488) -> (decimal integer string=w495:string)  [unwired: 1 in]
      n150 = Concatenate Strings("C", w495) -> (w494:string)
      n151 = while {
        tunnel: [w507] -> w501
        tunnel: [w506] -> w500
        tunnel: w494 -> [w505]
        tunnel: w493 -> [w504]
        tunnel: w492 -> [w503]
        stop <- TRUE stop-if-true
        n152 = VISA Write(VISA resource name=w504, write buffer=w505, error in (no error)=w503) -> (VISA resource name out=w507:refnum<visa-resource-name>, error out=w506:errorcluster)  [unwired: 1 out]
        n153 = Wait (ms)(milliseconds to wait=u32 10) -> ()  [unwired: 1 out]
      }
      n154 = property class="Instr"(reference=w501, error in=w500) -> (reference out=w498:refnum<visa-resource-name>, error out=w497:errorcluster, "Serial Settings:Number of Bytes at Serial Port"=w499:u32)
      n155 = VISA Read(VISA resource name=w498, byte count=w499, error in (no error)=w497) -> (VISA resource name out=w491:refnum<visa-resource-name>, read buffer=w489:string, error out=w490:errorcluster)  [unwired: 1 out]
    }
    frame "Set Low CO2 Alarm" {
      n156 = Number To Decimal String(number=w514) -> (decimal integer string=w516:string)  [unwired: 1 in]
      n157 = Concatenate Strings("L", w516) -> (w515:string)
      n158 = while {
        tunnel: [w528] -> w522
        tunnel: [w527] -> w521
        tunnel: w515 -> [w526]
        tunnel: w513 -> [w525]
        tunnel: w512 -> [w524]
        stop <- TRUE stop-if-true
        n159 = VISA Write(VISA resource name=w525, write buffer=w526, error in (no error)=w524) -> (VISA resource name out=w528:refnum<visa-resource-name>, error out=w527:errorcluster)  [unwired: 1 out]
        n160 = Wait (ms)(milliseconds to wait=u32 10) -> ()  [unwired: 1 out]
      }
      n161 = property class="Instr"(reference=w522, error in=w521) -> (reference out=w519:refnum<visa-resource-name>, error out=w518:errorcluster, "Serial Settings:Number of Bytes at Serial Port"=w520:u32)
      n162 = VISA Read(VISA resource name=w519, byte count=w520, error in (no error)=w518) -> (VISA resource name out=w511:refnum<visa-resource-name>, read buffer=w509:string, error out=w510:errorcluster)  [unwired: 1 out]
    }
    frame "Set Analog Output Type" {
      # "sending I0 sets voltage  0-5 V\nsending I1 sets current 4-20 mA"
      n163 = Number To Decimal String(number=w530) -> (decimal integer string=w537:string)  [unwired: 1 in]
      n164 = Concatenate Strings("I", w537) -> (w536:string)
      n165 = while {
        tunnel: [w549] -> w543
        tunnel: [w548] -> w542
        tunnel: w536 -> [w547]
        tunnel: w535 -> [w546]
        tunnel: w534 -> [w545]
        stop <- TRUE stop-if-true
        n166 = VISA Write(VISA resource name=w546, write buffer=w547, error in (no error)=w545) -> (VISA resource name out=w549:refnum<visa-resource-name>, error out=w548:errorcluster)  [unwired: 1 out]
        n167 = Wait (ms)(milliseconds to wait=u32 10) -> ()  [unwired: 1 out]
      }
      n168 = property class="Instr"(reference=w543, error in=w542) -> (reference out=w540:refnum<visa-resource-name>, error out=w539:errorcluster, "Serial Settings:Number of Bytes at Serial Port"=w541:u32)
      n169 = VISA Read(VISA resource name=w540, byte count=w541, error in (no error)=w539) -> (VISA resource name out=w533:refnum<visa-resource-name>, read buffer=w531:string, error out=w532:errorcluster)  [unwired: 1 out]
    }
    frame "Set Analog Output Scaling" {
      n170 = To Long Integer(number=w563) -> (32bit integer=w557:i32)
      n171 = Number To Decimal String(number=w556) -> (decimal integer string=w554:string)  [unwired: 1 in]
      n172 = Number To Decimal String(number=w557) -> (decimal integer string=w552:string)  [unwired: 1 in]
      n173 = Concatenate Strings("O", w554, ",", w552) -> (w551:string)
      n174 = while {
        tunnel: [w574] -> w568
        tunnel: [w573] -> w567
        tunnel: w562 -> [w572]
        tunnel: w561 -> [w571]
        tunnel: w551 -> [w570]
        stop <- TRUE stop-if-true
        n175 = VISA Write(VISA resource name=w572, write buffer=w570, error in (no error)=w571) -> (VISA resource name out=w574:refnum<visa-resource-name>, error out=w573:errorcluster)  [unwired: 1 out]
        n176 = Wait (ms)(milliseconds to wait=u32 10) -> ()  [unwired: 1 out]
      }
      n177 = property class="Instr"(reference=w568, error in=w567) -> (reference out=w565:refnum<visa-resource-name>, error out=w564:errorcluster, "Serial Settings:Number of Bytes at Serial Port"=w566:u32)
      n178 = VISA Read(VISA resource name=w565, byte count=w566, error in (no error)=w564) -> (VISA resource name out=w560:refnum<visa-resource-name>, read buffer=w558:string, error out=w559:errorcluster)  [unwired: 1 out]
    }
    frame "Set Data Valid Pin I/O" {
      # "J0 sets datavalid mode\nJ1 sets analog input mode"
      n179 = Number To Decimal String(number=w581) -> (decimal integer string=w583:string)  [unwired: 1 in]
      n180 = Concatenate Strings("J", w583) -> (w582:string)
      n181 = while {
        tunnel: [w596] -> w589
        tunnel: [w595] -> w588
        tunnel: w582 -> [w594]
        tunnel: w580 -> [w593]
        tunnel: w579 -> [w592]
        stop <- TRUE stop-if-true
        n182 = VISA Write(VISA resource name=w593, write buffer=w594, error in (no error)=w592) -> (VISA resource name out=w596:refnum<visa-resource-name>, error out=w595:errorcluster)  [unwired: 1 out]
        n183 = Wait (ms)(milliseconds to wait=u32 10) -> ()  [unwired: 1 out]
      }
      n184 = property class="Instr"(reference=w589, error in=w588) -> (reference out=w586:refnum<visa-resource-name>, error out=w585:errorcluster, "Serial Settings:Number of Bytes at Serial Port"=w587:u32)
      n185 = VISA Read(VISA resource name=w586, byte count=w587, error in (no error)=w585) -> (VISA resource name out=w578:refnum<visa-resource-name>, read buffer=w576:string, error out=w577:errorcluster)  [unwired: 1 out]
    }
    frame "Save Current Settings" {
      n186 = while {
        tunnel: [w613] -> w607
        tunnel: [w612] -> w606
        tunnel: w602 -> [w611]
        tunnel: w601 -> [w610]
        tunnel: "X" -> [w609]
        stop <- TRUE stop-if-true
        n187 = VISA Write(VISA resource name=w611, write buffer=w609, error in (no error)=w610) -> (VISA resource name out=w613:refnum<visa-resource-name>, error out=w612:errorcluster)  [unwired: 1 out]
        n188 = Wait (ms)(milliseconds to wait=u32 10) -> ()  [unwired: 1 out]
      }
      n189 = property class="Instr"(reference=w607, error in=w606) -> (reference out=w604:refnum<visa-resource-name>, error out=w603:errorcluster, "Serial Settings:Number of Bytes at Serial Port"=w605:u32)
      n190 = VISA Read(VISA resource name=w604, byte count=w605, error in (no error)=w603) -> (VISA resource name out=w600:refnum<visa-resource-name>, read buffer=w599:string, error out=w598:errorcluster)  [unwired: 1 out]
    }
    frame "Restore Default Settings" {
      n191 = while {
        tunnel: [w631] -> w625
        tunnel: [w630] -> w624
        tunnel: "]" -> [w629]
        tunnel: w619 -> [w628]
        tunnel: w618 -> [w627]
        stop <- TRUE stop-if-true
        n192 = VISA Write(VISA resource name=w628, write buffer=w629, error in (no error)=w627) -> (VISA resource name out=w631:refnum<visa-resource-name>, error out=w630:errorcluster)  [unwired: 1 out]
        n193 = Wait (ms)(milliseconds to wait=u32 10) -> ()  [unwired: 1 out]
      }
      n194 = property class="Instr"(reference=w625, error in=w624) -> (reference out=w622:refnum<visa-resource-name>, error out=w621:errorcluster, "Serial Settings:Number of Bytes at Serial Port"=w623:u32)
      n195 = VISA Read(VISA resource name=w622, byte count=w623, error in (no error)=w621) -> (VISA resource name out=w617:refnum<visa-resource-name>, read buffer=w615:string, error out=w616:errorcluster)  [unwired: 1 out]
    }
    frame "Display Current Settings" {
      n196 = while {
        tunnel: [w649] -> w643
        tunnel: [w648] -> w642
        tunnel: "?" -> [w647]
        tunnel: w637 -> [w646]
        tunnel: w636 -> [w645]
        stop <- TRUE stop-if-true
        n197 = VISA Write(VISA resource name=w646, write buffer=w647, error in (no error)=w645) -> (VISA resource name out=w649:refnum<visa-resource-name>, error out=w648:errorcluster)  [unwired: 1 out]
        n198 = Wait (ms)(milliseconds to wait=u32 10) -> ()  [unwired: 1 out]
      }
      n199 = property class="Instr"(reference=w643, error in=w642) -> (reference out=w640:refnum<visa-resource-name>, error out=w639:errorcluster, "Serial Settings:Number of Bytes at Serial Port"=w641:u32)
      n200 = VISA Read(VISA resource name=w640, byte count=w641, error in (no error)=w639) -> (VISA resource name out=w635:refnum<visa-resource-name>, read buffer=w633:string, error out=w634:errorcluster)  [unwired: 1 out]
    }
    frame "Zero" {
      n201 = while {
        tunnel: [w668] -> w660
        tunnel: [w667] -> w659
        tunnel: w652 -> [w664]
        tunnel: w651 -> [w663]
        stop <- TRUE stop-if-true
        n202 = Wait (ms)(milliseconds to wait=u32 20000) -> ()  [unwired: 1 out]
        n203 = VISA Write(VISA resource name=w664, write buffer="Z", error in (no error)=w663) -> (VISA resource name out=w668:refnum<visa-resource-name>, error out=w667:errorcluster)  [unwired: 1 out]
      }
      n204 = property class="Instr"(reference=w660, error in=w659) -> (reference out=w656:refnum<visa-resource-name>, error out=w657:errorcluster, "Serial Settings:Number of Bytes at Serial Port"=w658:u32)
      n205 = VISA Read(VISA resource name=w656, byte count=w658, error in (no error)=w657) -> (VISA resource name out=w662:refnum<visa-resource-name>, read buffer=w655:string, error out=w661:errorcluster)  [unwired: 1 out]
      n206 = VISA Flush I/O Buffer(VISA resource name=w662, error in (no error)=w661) -> (VISA resource name out=w653:refnum<visa-resource-name>, error out=w654:errorcluster)  [unwired: 1 in]
    }
    frame "Time" {
      n207 = VISA Clear(VISA resource name=w675, error in (no error)=w674) -> (VISA resource name out=w677:refnum<visa-resource-name>, error out=w676:errorcluster)
      n208 = while {
        tunnel: [w688] -> w673
        tunnel: [w687] -> w671
        tunnel: [w686] -> w672
        tunnel: w677 -> [w680]
        tunnel: w676 -> [w679]
        tunnel: [w678] -> w670
        i -> [w683]
        stop <- w685 stop-if-true
        n209 = flat-sequence {
          tunnel: [w714] -> w694
          tunnel: [w713] -> w693
          tunnel: w680 -> [w712]
          tunnel: w679 -> [w711]
          frame #0 {
            n210 = Wait (ms)(milliseconds to wait=u32 200) -> ()  [unwired: 1 out]
            n211 = VISA Write(VISA resource name=w712, write buffer="##time$$", error in (no error)=w711) -> (VISA resource name out=w714:refnum<visa-resource-name>, error out=w713:errorcluster)  [unwired: 1 out]
          }
        }
        n212 = property class="Instr"(reference=w694, error in=w693) -> (reference out=w691:refnum<visa-resource-name>, error out=w690:errorcluster, "Serial Settings:Number of Bytes at Serial Port"=w689:u32)
        n213 = Greater Than 0?(x=w689) -> (x > 0?=w692:bool)
        n214 = case shown="True" w692 {
          tunnel: w691 -> [w698 w710]
          tunnel: w690 -> [w697 w709]
          tunnel: w689 -> [w696 w708]
          tunnel: [FALSE w704] -> w684
          tunnel: [w698 w707] -> w688
          tunnel: [w697 w706] -> w687
          tunnel: [w696 w699] -> w686
          tunnel: [_ w701] -> w678
          frame False {
          }
          frame True {
            w705 = T2 16 items=["Flush Receive Buffer"=16, "Write Transmit Buffer to Device"=32, "Flush Receive Buffer (No I/O)"=64, "Flush Transmit Buffer"=128] ("Mask")
            n215 = VISA Read(VISA resource name=w710, byte count=w708, error in (no error)=w709) -> (VISA resource name out=w703:refnum<visa-resource-name>, read buffer=w701:string, error out=w702:errorcluster)  [unwired: 1 out]
            n216 = Fract/Exp String To Number(string=w701) -> (number=w700:dbl)  [unwired: 3 in, 1 out]
            n217 = To Long Integer(number=w700) -> (32bit integer=w699:i32)
            n218 = Not Equal To 0?(x=w700) -> (x != 0?=w704:bool)
            n219 = VISA Flush I/O Buffer(VISA resource name=w703, mask (16)=w705, error in (no error)=w702) -> (VISA resource name out=w707:refnum<visa-resource-name>, error out=w706:errorcluster)
          }
        }
        n220 = Greater?(x=w683, y=4) -> (0:w681:bool)
        n221 = Or(x=w684, y=w681) -> (x .or. y?=w685:bool)
      }
    }
  }
  "StringFromSBA-5" <- w5
  "error out" <- w3
  "dup VISA resource name" <- w4
  "bytes out" <- w2
